vi "Get Default Data from TD--WithTIMESTAMP.vi"(8 "error in":errorcluster, 10 "Type Descriptor":T1) -> (0 "error out":errorcluster, 2 "Default VData":variant)   [LabVIEW 2011]
doc: "Returns default data of the type defined by the TD. This vi calls itself recursively."
uses:
  <userlib>/_OpenG.lib/lvdata/lvdata.llb/Type Descriptor__ogtk.ctl
panel:
  in  "for recursive call to self":refnum<vi>
  # "[OpenG VI Tags] ***Do Not Remove***\nSVN Revision = 659\nSVN Revision Date = 2006-12-02 11:58:44 -0800 (Sat, 02 Dec 2006)\nPackage = oglib_lvdata-2.8-1\nDepends = oglib_error-2.0-1"
  # "Get Default Data from TD.vi\n\nReturns default data of the type defined by the TD.  This vi calls itself recurs\n\nPlease visit http://www.OpenG.org to learn about the\nOpen Source LabVIEW software movement.\n\nNOTICE -- YOU MUST LEAVE THIS NOTICE IN PLACE.  PER THE TERMS OF THE LICENSE BELOW, YOU MAY SUBLICENSE THIS SOFTWARE \nIN ANY WAY THAT DOES NOT CONFLICT WITH THIS LICENSE.\n\n### BSD License (http://www.opensource.org/licenses/bsd-license.php) Begin ###\n \nCopyright (c) 2002, Jean-Pierre Drolet <drolet_jp@hotmail.com>\nCopyright (c) 2002-2006, Jim Kring <jim@jimkring.com>\n\nAll rights reserved.\n\nRedistribution and use in source and binary forms, with or without modification, are permitted provided that the following conditions are met:\n\n    * Redistributions of source code must retain the above copyright notice, this list of conditions and the following disclaimer.\n    * Redistributions in binary form must reproduce the above copyright notice, this list of conditions and the following disclaimer in the \n       documentation and/or other materials provided with the distribution.\n    * Neither the name of SciWare, James Kring, Inc., nor the names of its contributors may be used to endorse or promote products derived \n       from this software without specific prior written permission.\n\nTHIS SOFTWARE IS PROVIDED BY THE COPYRIGHT HOLDERS AND CONTRIBUTORS \"AS IS\" AND ANY EXPRESS OR IMPLIED WARRANTIES, \nINCLUDING, BUT NOT LIMITED TO, THE IMPLIED WARRANTIES OF MERCHANTABILITY AND FITNESS FOR A PARTICULAR PURPOSE ARE \nDISCLAIMED. IN NO EVENT SHALL THE COPYRIGHT OWNER OR CONTRIBUTORS BE LIABLE FOR ANY DIRECT, INDIRECT, INCIDENTAL,\n SPECIAL, EXEMPLARY, OR CONSEQUENTIAL DAMAGES (INCLUDING, BUT NOT LIMITED TO, PROCUREMENT OF SUBSTITUTE GOODS OR \nSERVICES; LOSS OF USE, DATA, OR PROFITS; OR BUSINESS INTERRUPTION) HOWEVER CAUSED AND ON ANY THEORY OF LIABILITY, \nWHETHER IN CONTRACT, STRICT LIABILITY, OR TORT (INCLUDING NEGLIGENCE OR OTHERWISE) ARISING IN ANY WAY OUT OF THE USE \nOF THIS SOFTWARE, EVEN IF ADVISED OF THE POSSIBILITY OF SUCH DAMAGE.\n\n### BSD License End ###"
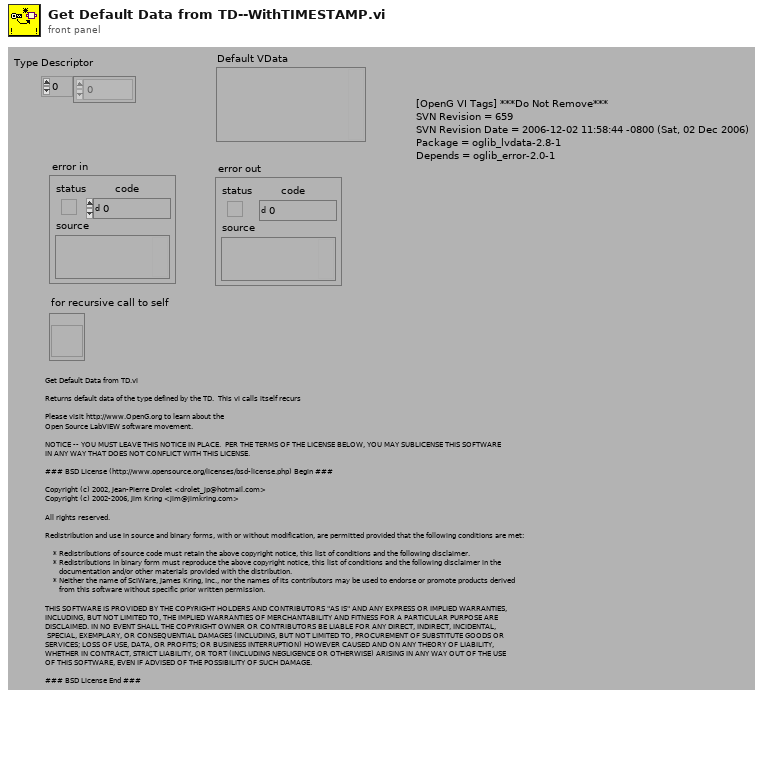
[diagram p1: front panel]
types:
  T1 = typedef "Type Descriptor__ogtk.ctl" = i16[]
  T2 = typedef "Type Descriptor Header__ogtk.ctl" = cluster{"length":u16, "private":u8, "type":T3, "# elements":u16}
  T3 = typedef "Type Descriptor Enumeration__ogtk.ctl" = enum8{"<Null>", "I8", "I16", "I32", "I64", "U8", "U16", "U32", "U64", "SGL", "DBL", "EXT", "CSG", "CDB", "CXT", "0x0F", "0x10", "0x11", "0x12", "0x13", "0x14", "Enum U8", "Enum U16", "Enum U32", "Enum U64", "SGL PQ", "DBL PQ", "EXT PQ", "CSG PQ", "CDB PQ", "CXT PQ", "0x1F", "0x20", "Boolean", "0x22", "0x23", "0x24", "0x25", "0x26", "0x27", "0x28", "0x29", "0x2A", "0x2B", "0x2C", "0x2D", "0x2E", "0x2F", "String", "0x31", "Path", "Pict", "0x34", "0x35", "0x36", "DAQ", "0x38", "0x39", "0x3A", "0x3B", "0x3C", "0x3D", "0x3E", "0x3F", "Array", "0x41", "0x42", "0x43", "0x44", "0x45", "0x46", "0x47", "0x48", "0x49", "0x4A", "0x4B", "0x4C", "0x4D", "0x4E", "0x4F", "Cluster", "0x51", "0x52", "Variant", "Waveform", "0x55", "0x56", "0x57", "0x58", "0x59", "0x5A", "0x5B", "0x5C", "0x5D", "0x5E", "0x5F", "0x60", "0x61", "0x62", "0x63", "0x64", "0x65", "0x66", "0x67", "0x68", "0x69", "0x6A", "0x6B", "0x6C", "0x6D", "0x6E", "0x6F", "Refnum"}
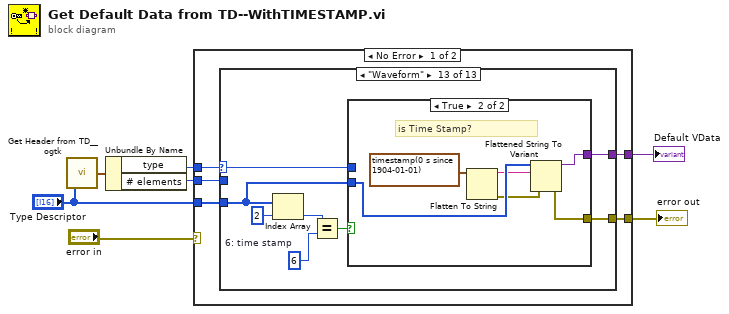
[diagram p0: block diagram]
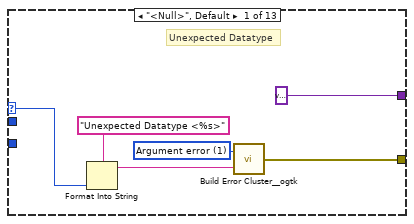
[diagram p2: hidden frame]
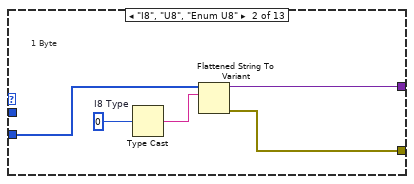
[diagram p3: hidden frame]
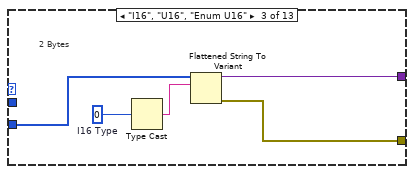
[diagram p4: hidden frame]
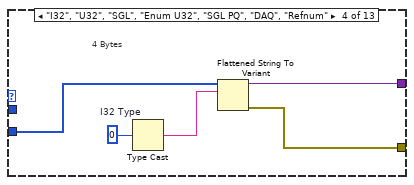
[diagram p5: hidden frame]
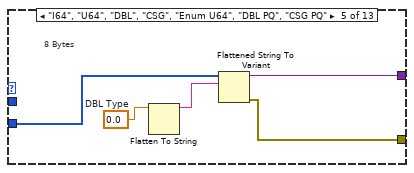
[diagram p6: hidden frame]
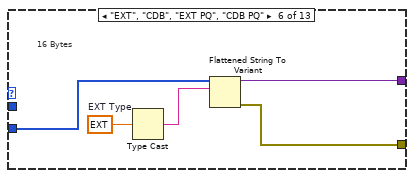
[diagram p7: hidden frame]
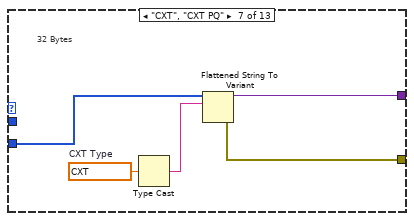
[diagram p8: hidden frame]
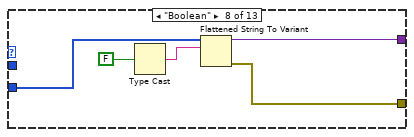
[diagram p9: hidden frame]
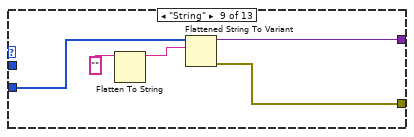
[diagram p10: hidden frame]
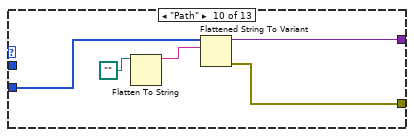
[diagram p11: hidden frame]
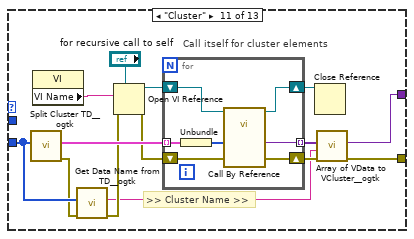
[diagram p12: hidden frame]
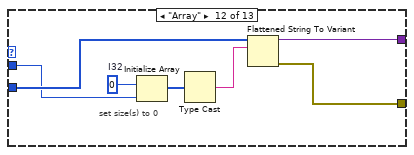
[diagram p13: hidden frame]
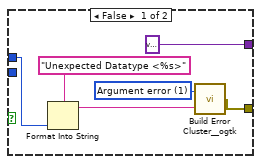
[diagram p14: hidden frame]
diagram:
  n1 = call <userlib>:"Get Header from TD__ogtk.vi"("Type Descriptor"="Type Descriptor") -> ("Type Descriptor Header"=w3:T2)
  n2 = Unbundle By Name(w3) -> ("type"=w2:T3, "# elements"=w1:u16)
  n3 = case shown="No Error" "error in" {
    selector: "error in" -> [_ w113]
    tunnel: w2 -> [w12 _]
    tunnel: [w11 w113] -> w5
    tunnel: "Type Descriptor" -> [w10 _]
    tunnel: [w9 variant] -> w4
    tunnel: w1 -> [w8 _]
    frame No Error {
      n4 = case shown="\"Waveform\"" w12 {
        selector: w12 -> [w15 _ _ _ _ _ _ _ _ _ _ _ w93]
        tunnel: [w14 w19 w26 w29 w35 w40 w46 w51 w54 w59 w64 w90 w94] -> w11
        tunnel: w10 -> [_ w21 w27 w31 w36 w42 w45 w52 w56 w62 w69 w89 w92]
        tunnel: [variant w20 w25 w30 w34 w39 w44 w49 w55 w60 w65 w91 w98] -> w9
        tunnel: w8 -> [_ _ _ _ _ _ _ _ _ _ _ w85 _]
        frame "<Null>", Default {
          w16 = 1 items=["No error", "Argument error", "Memory is full", "Out of zone", "End of file", "File already open", "Generic file I/O error", "File not found", "File permission error", "Disk is full", "Duplicate path", "Too many files open", "System feature not enabled", "Resource file not found", "Cannot add resource", "Resource not found", "Image not found", "Image memory error", "Pen does not exist", "Config type invalid", "Config token not found", "Config parse error", "Config memory error", "Bad external code format", "Bad external code offset", "External code not present", "Null window", "Destroy window error", "Null menu", "Print aborted", "Bad print record", "Print driver error", "Windows error during printing", "Memory error during printing", "Print dialog error", "Generic print error", "Invalid device refnum", "Device not found", "Device parameter error", "Device unit error", "Cannot open device", "Device call aborted", "Generic error", "Cancelled by user", "Object ID too low", "Object ID too high", "Object not in heap", "Unknown heap", "Unknown object (invalid DefProc)", "Unknown object (DefProc not in table)", "Message out of range", "Invalid (null) method", "Unknown message", "Manager call not supported", "Bad address", "Network operation in progress", "Network operation timed out", "Connection is busy", "Network attribute not supported", "Network error", "Address in use", "System out of memory", "Connection aborted", "Connection refused", "Not connected", "Already connected", "Connection closed", "Initialization error (interapplication manager)", "Bad occurrence", "Wait on unbound occurrence handler", "Occurrence queue overflow", "Datalog type conflict", "Unused", "Unrecognized type (interapplication manager)", "Memory corrupt", "Failed to make temporary DLL", "Old CIN version", "Drag socket not found", "Failed to load drop-object", "Failed to register OLE object", "Failed to release OLE object", "Format specifier type mismatch", "Unknown format specifier", "Too few format specifiers", "Too many format specifiers", "Scan failed", "Newer CIN version", "Error converting to variant", "Runtime menu error", "Password tampered", "Variant attribute not found", "Incompatible variant data type", "Event data is not available", "Event Store is not present", "Occurrence is not found", "Event Queue is not created", "Event info is not available", "Refnum passed is NULL", "Error retrieving Class GUID", "Error retrieving CoClass GUID", "Error retrieving TypeLib GUID.", "Bad built application magic bytes.", "Specific driver is different from the specific driver associated with the Logical Name.", "There is no session opened to the class driver.", "Max Error", "MAX - Error with config objects", "MAX - Error loading configuration", "MAX - Group not supported"]
          # "Unexpected Datatype"
          n5 = Format Into String(format string="Unexpected Datatype <%s>" ("Format String"), w15) -> (resulting string=w18:string)  [unwired: 2 in, 1 out]
          n6 = call <userlib>:"Build Error Cluster__ogtk.vi"("String to Prepend to source (\"\")"=w18, "code"=w16) -> ("error out"=w14:errorcluster)
        }
        frame "I8", "U8", "Enum U8" {
          w23 = i8 0  # I8 Type
          # "1 Byte"
          n7 = Type Cast(x=w23) -> (*(type *) &x=w22:string)  [unwired: 1 in]
          n8 = Flattened String To Variant(6:w22, 7:w21) -> (0:w19:errorcluster, 3:w20:variant)  [unwired: 1 in]
        }
        frame "I16", "U16", "Enum U16" {
          w28 = i16 0  # I16 Type
          # "2 Bytes"
          n9 = Type Cast(x=w28) -> (*(type *) &x=w24:string)  [unwired: 1 in]
          n10 = Flattened String To Variant(6:w24, 7:w27) -> (0:w26:errorcluster, 3:w25:variant)  [unwired: 1 in]
        }
        frame "I32", "U32", "SGL", "Enum U32", "SGL PQ", "DAQ", "Refnum" {
          w33 = 0  # I32 Type
          # "4 Bytes"
          n11 = Type Cast(x=w33) -> (*(type *) &x=w32:string)  [unwired: 1 in]
          n12 = Flattened String To Variant(6:w32, 7:w31) -> (0:w29:errorcluster, 3:w30:variant)  [unwired: 1 in]
        }
        frame "I64", "U64", "DBL", "CSG", "Enum U64", "DBL PQ", "CSG PQ" {
          w38 = 0.0  # DBL Type
          # "8 Bytes"
          n13 = Flatten To String(anything=w38) -> (data string=w37:string)  [unwired: 3 in, 2 out]
          n14 = Flattened String To Variant(6:w37, 7:w36) -> (0:w35:errorcluster, 3:w34:variant)  [unwired: 1 in]
        }
        frame "EXT", "CDB", "EXT PQ", "CDB PQ" {
          w43 = ext 0.0  # EXT Type
          # "16 Bytes"
          n15 = Type Cast(x=w43) -> (*(type *) &x=w41:string)  [unwired: 1 in]
          n16 = Flattened String To Variant(6:w41, 7:w42) -> (0:w40:errorcluster, 3:w39:variant)  [unwired: 1 in]
        }
        frame "CXT", "CXT PQ" {
          w48 = cxt 0.0+0.0i  # CXT Type
          # "32 Bytes"
          n17 = Type Cast(x=w48) -> (*(type *) &x=w47:string)  [unwired: 1 in]
          n18 = Flattened String To Variant(6:w47, 7:w45) -> (0:w46:errorcluster, 3:w44:variant)  [unwired: 1 in]
        }
        frame "Boolean" {
          n19 = Type Cast(x=FALSE ("status")) -> (*(type *) &x=w50:string)  [unwired: 1 in]
          n20 = Flattened String To Variant(6:w50, 7:w52) -> (0:w51:errorcluster, 3:w49:variant)  [unwired: 1 in]
        }
        frame "String" {
          n21 = Flatten To String(anything="") -> (data string=w57:string)  [unwired: 3 in, 2 out]
          n22 = Flattened String To Variant(6:w57, 7:w56) -> (0:w54:errorcluster, 3:w55:variant)  [unwired: 1 in]
        }
        frame "Path" {
          n23 = Flatten To String(anything=path "") -> (data string=w61:string)  [unwired: 3 in, 2 out]
          n24 = Flattened String To Variant(6:w61, 7:w62) -> (0:w59:errorcluster, 3:w60:variant)  [unwired: 1 in]
        }
        frame "Cluster" {
          # ">> Cluster Name >>"
          # "Call itself for cluster elements"
          n25 = call <userlib>:"Split Cluster TD__ogtk.vi"("Type Descriptor"=w69) -> ("error out"=w68:errorcluster, "Type Descriptors"=w76:cluster{"Type Descriptor":T1}[])  [unwired: 9 in]
          n26 = property class="VI"() -> ("VI Name"=w74:string)  [unwired: 2 in, 2 out]
          n27 = call <userlib>:"Get Data Name from TD__ogtk.vi"("error in (no error)"=w68, "Type Descriptor"=w69) -> ("error"=w67:errorcluster, "name"=w66:string)  [unwired: 8 in]
          n28 = Open VI Reference(type specifier VI Refnum (for type only)="for recursive call to self", vi path=w74, error in (no error)=w67) -> (vi reference=w73:refnum<vi>, error out=w70:errorcluster)  [unwired: 3 in]
          n29 = for {
            tunnel: w76 -> [w84] mode=indexing
            shift-right: [w81] -> w71
            shift-left: w70 -> [w82]
            tunnel: [w80] -> w77 mode=indexing
            shift-right: [w78] -> w72
            shift-left: w73 -> [w79]
            n30 = Unbundle(w84) -> ("Type Descriptor"=w83:T1)
            n31 = call-by-ref "?"(reference=w79, "error in"=w82, "type string"=w83) -> (reference out=w78:refnum<vi>, "error out"=w81:errorcluster, "Default VData"=w80:variant)  [unwired: 9 in, 1 out]
          }
          n32 = Close Reference(reference=w72) -> ()  [unwired: 1 in, 1 out]
          n33 = call <userlib>:"Array of VData to VCluster__ogtk.vi"("error in (no error)"=w71, "Cluster Name"=w66, "Array"=w77) -> ("error out"=w64:errorcluster, "VCluster"=w65:variant)  [unwired: 7 in]
        }
        frame "Array" {
          w88 = 0  # I32
          # "set size(s) to 0"
          n34 = Initialize Array(w88, w85) -> (w87:i32[])
          n35 = Type Cast(x=w87) -> (*(type *) &x=w86:string)  [unwired: 1 in]
          n36 = Flattened String To Variant(6:w86, 7:w89) -> (0:w90:errorcluster, 3:w91:variant)  [unwired: 1 in]
        }
        frame "Waveform" {
          w96 = i16 6  # 6: time stamp
          n37 = Index Array(array=w92, index=2) -> (element=w97:i16)
          n38 = Equal?(x=w97, y=w96) -> (x = y?=w95:bool)
          n39 = case shown="True" w95 {
            tunnel: [variant ("Default VData") w110] -> w98
            tunnel: [w101 w109] -> w94
            tunnel: w93 -> [w100 _]
            tunnel: w92 -> [_ w111]
            frame False {
              w102 = 1 items=["No error", "Argument error", "Memory is full", "Out of zone", "End of file", "File already open", "Generic file I/O error", "File not found", "File permission error", "Disk is full", "Duplicate path", "Too many files open", "System feature not enabled", "Resource file not found", "Cannot add resource", "Resource not found", "Image not found", "Image memory error", "Pen does not exist", "Config type invalid", "Config token not found", "Config parse error", "Config memory error", "Bad external code format", "Bad external code offset", "External code not present", "Null window", "Destroy window error", "Null menu", "Print aborted", "Bad print record", "Print driver error", "Windows error during printing", "Memory error during printing", "Print dialog error", "Generic print error", "Invalid device refnum", "Device not found", "Device parameter error", "Device unit error", "Cannot open device", "Device call aborted", "Generic error", "Cancelled by user", "Object ID too low", "Object ID too high", "Object not in heap", "Unknown heap", "Unknown object (invalid DefProc)", "Unknown object (DefProc not in table)", "Message out of range", "Invalid (null) method", "Unknown message", "Manager call not supported", "Bad address", "Network operation in progress", "Network operation timed out", "Connection is busy", "Network attribute not supported", "Network error", "Address in use", "System out of memory", "Connection aborted", "Connection refused", "Not connected", "Already connected", "Connection closed", "Initialization error (interapplication manager)", "Bad occurrence", "Wait on unbound occurrence handler", "Occurrence queue overflow", "Datalog type conflict", "Unused", "Unrecognized type (interapplication manager)", "Memory corrupt", "Failed to make temporary DLL", "Old CIN version", "Drag socket not found", "Failed to load drop-object", "Failed to register OLE object", "Failed to release OLE object", "Format specifier type mismatch", "Unknown format specifier", "Too few format specifiers", "Too many format specifiers", "Scan failed", "Newer CIN version", "Error converting to variant", "Runtime menu error", "Password tampered", "Variant attribute not found", "Incompatible variant data type", "Event data is not available", "Event Store is not present", "Occurrence is not found", "Event Queue is not created", "Event info is not available", "Refnum passed is NULL", "Error retrieving Class GUID", "Error retrieving CoClass GUID", "Error retrieving TypeLib GUID.", "Bad built application magic bytes.", "Specific driver is different from the specific driver associated with the Logical Name.", "There is no session opened to the class driver.", "Max Error", "MAX - Error with config objects", "MAX - Error loading configuration", "MAX - Group not supported"]
              n40 = Format Into String(format string="Unexpected Datatype <%s>" ("Format String"), w100) -> (resulting string=w104:string)  [unwired: 2 in, 1 out]
              n41 = call <userlib>:"Build Error Cluster__ogtk.vi"("String to Prepend to source (\"\")"=w104, "code"=w102) -> ("error out"=w101:errorcluster)
            }
            frame True {
              # "is Time Stamp?"
              n42 = Flatten To String(anything=timestamp(0 s since 1904-01-01)) -> (data string=w107:string, error out=w106:errorcluster)  [unwired: 3 in, 1 out]
              n43 = Flattened String To Variant(4:w106, 6:w107, 7:w111) -> (0:w109:errorcluster, 3:w110:variant)
            }
          }
        }
      }
    }
    frame Error {
    }
  }
  "error out" <- w5
  "Default VData" <- w4
